vi "Auto-Approach_mod.vi"(6 "Error in":errorcluster, 7 "max steps":i32=5555555, 8 "Wait for motor (ms)":u32=50, 9 "Application reference":refnum<vi>) -> (0 "error out":errorcluster, 1 "Surface reached":bool, 2 "steps taken":i32, 3 "Application ref out":refnum<vi>)   [LabVIEW 2019]
doc: "Programming Interface Example: Automatic approach implemented using Nanonis Programming Interface functions. This can be used if you want to execute special functions after each motor step or if you want to control your motor directly from LabVIEW.\n\n- Nanonis Programming Interface -"
panel:
  in  "stop":bool
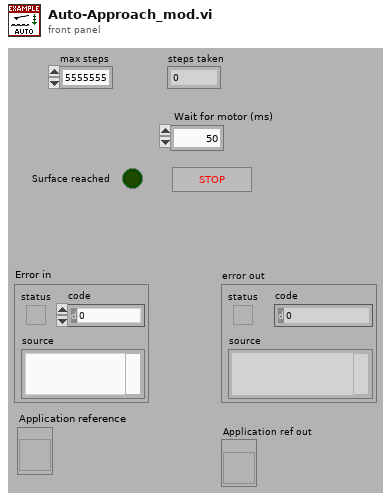
[diagram p1: front panel]
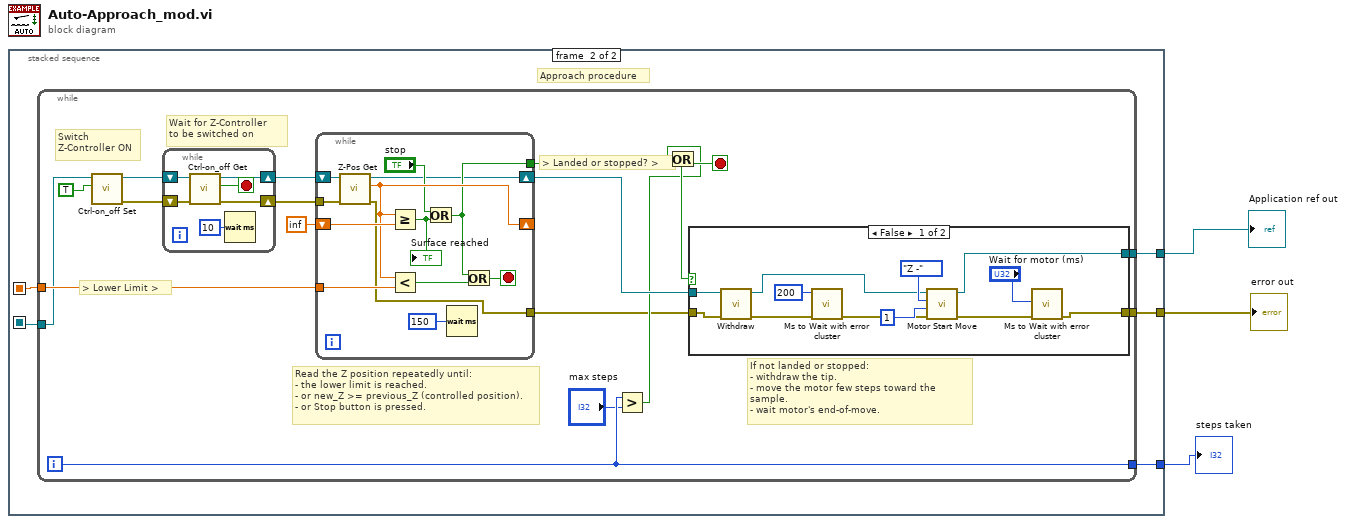
[diagram p0: block diagram]
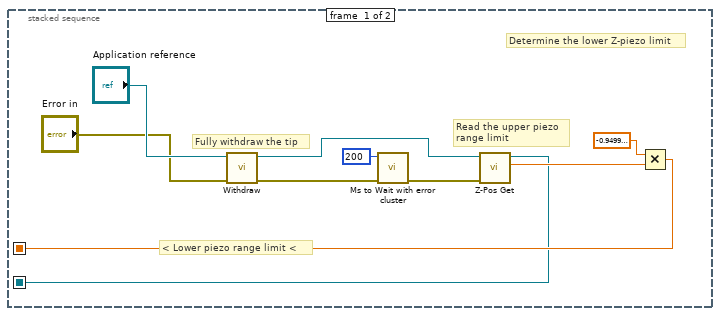
[diagram p2: hidden frame]
diagram:
  n1 = stacked-sequence {
    seq-local: [w12 _] -> [_ w18]
    seq-local: [w7 _] -> [_ w17]
    tunnel: [_ w16] -> w3
    tunnel: [_ w15] -> w2
    tunnel: [_ w14] -> w1
    frame #0 {
      # "Read the upper piezo\nrange limit"
      # "Fully withdraw the tip"
      # "< Lower piezo range limit <"
      # "Determine the lower Z-piezo limit"
      n2 = call <userlib>:"Withdraw.vi"("Error in (no error)"="Error in", "Application ref in"="Application reference") -> ("Error out"=w9:errorcluster, "Application ref out"=w6:refnum<vi>)  [unwired: 8 in]
      n3 = call <userlib>:"Ms to Wait with error cluster.vi"("error in (no error)"=w9, "milliseconds to wait"=u32 200) -> ("error out"=w8:errorcluster)  [unwired: 4 in, 1 out]
      n4 = call <userlib>:"Z-Pos Get.vi"("error in (no error)"=w8, "Application ref in"=w6) -> ("Z position (m)"=w11:sgl, "Application ref out"=w7:refnum<vi>)  [unwired: 7 in, 1 out]
      n5 = Multiply(x=sgl -0.95, y=w11) -> (x*y=w12:sgl)
    }
    frame #1 {
      # "Approach procedure"
      n6 = while {
        tunnel: w18 -> [w35]
        tunnel: w17 -> [w30]
        tunnel: [w23] -> w16
        tunnel: [w21] -> w15
        tunnel: [w20] -> w14
        i -> [w23]
        stop <- w25 stop-if-true
        # "Wait for Z-Controller\nto be switched on"
        # "> Lower Limit >"
        # "Switch Z-Controller ON"
        # "> Landed or stopped? >"
        # "Read the Z position repeatedly until:\n- the lower limit is reached.\n- or new_Z >= previous_Z (controlled position).\n- or Stop button is pressed."
        # "If not landed or stopped:\n- withdraw the tip.\n- move the motor few steps toward the sample.\n- wait motor's end-of-move."
        n7 = call <userlib>:"Ctrl-on_off Set.vi"("Z Controller ON/OFF"=TRUE ("Ctrl on/off"), "Application ref in"=w30) -> ("error out"=w32:errorcluster, "Application ref out"=w29:refnum<vi>)  [unwired: 8 in]
        n8 = while {
          shift-right: [w41] -> w31
          shift-left: w32 -> [w40]
          shift-right: [w36] -> w28
          shift-left: w29 -> [w37]
          stop <- w39 stop-if-true
          n9 = call <userlib>:"Ctrl-on_off Get.vi"("error in (no error)"=w40, "Application ref in"=w37) -> ("error out"=w41:errorcluster, "Z-Controller on/off status"=w39:bool, "Application ref out"=w36:refnum<vi>)  [unwired: 7 in]
          n10 = Wait (ms)(milliseconds to wait=u32 10) -> ()  [unwired: 1 out]
        }
        n11 = while {
          shift-right: [w52] -> _
          shift-left: sgl inf ("Z-pos (m)") -> [w54]
          tunnel: [w48] -> w26
          tunnel: w35 -> [w46]
          tunnel: w31 -> [w45]
          shift-right: [w43] -> w27
          shift-left: w28 -> [w44]
          tunnel: [w42] -> w19
          stop <- w49 stop-if-true
          n12 = call <userlib>:"Z-Pos Get.vi"("error in (no error)"=w45, "Application ref in"=w44) -> ("error out"=w42:errorcluster, "Z position (m)"=w52:sgl, "Application ref out"=w43:refnum<vi>)  [unwired: 7 in]
          n13 = Greater Or Equal?(x=w52, y=w54) -> (x >= y?=w51:bool)
          "Surface reached" <- w51
          n14 = Less?(x=w52, y=w46) -> (x < y?=w50:bool)
          n15 = Or(x="stop", y=w51) -> (x .or. y?=w48:bool)
          n16 = Wait (ms)(milliseconds to wait=u32 150) -> ()  [unwired: 1 out]
          n17 = Or(x=w48, y=w50) -> (x .or. y?=w49:bool)
        }
        n18 = Greater?(x=w23, y="max steps") -> (0:w24:bool)
        n19 = Or(x=w24, y=w26) -> (x .or. y?=w25:bool)
        n20 = case shown="False" w26 {
          tunnel: w27 -> [w59 w68]
          tunnel: [w57 w67] -> w21
          tunnel: [w56 w68] -> w20
          tunnel: w19 -> [w55 w67]
          frame False {
            n21 = call <userlib>:"Withdraw.vi"("Error in (no error)"=w55, "Application ref in"=w59) -> ("Error out"=w64:errorcluster, "Application ref out"=w58:refnum<vi>)  [unwired: 8 in]
            n22 = call <userlib>:"Ms to Wait with error cluster.vi"("error in (no error)"=w64, "milliseconds to wait"=u32 200) -> ("error out"=w63:errorcluster)  [unwired: 4 in, 1 out]
            n23 = call <userlib>:"Motor Start Move.vi"("Error in (no error)"=w63, "Number of steps"=u16 1 ("Motor steps"), "Direction"=enum16{"X +", "X -", "Y +", "Y -", "Z +", "Z -"}."Z -", "Application ref in"=w58) -> ("Error out"=w61:errorcluster, "Application ref out"=w56:refnum<vi>)  [unwired: 5 in]
            n24 = call <userlib>:"Ms to Wait with error cluster.vi"("error in (no error)"=w61, "milliseconds to wait"="Wait for motor (ms)") -> ("error out"=w57:errorcluster)  [unwired: 4 in, 1 out]
          }
          frame True {
          }
        }
      }
    }
  }
  "steps taken" <- w3
  "error out" <- w2
  "Application ref out" <- w1
